vi "Setup - Forrmat Variant Into String.vi"(8 "error in (no error)":errorcluster) -> (0 "error out":errorcluster, 2 "Input String":string, 3 "Refnum":refnum<file>)   [LabVIEW 2009]
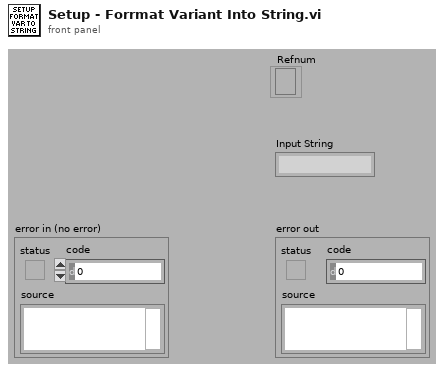
[diagram p1: front panel]
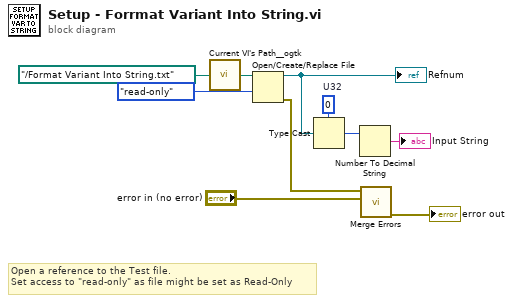
[diagram p0: block diagram]
diagram:
  w7 = u32 0  # U32
  # "Open a reference to the Test file.\nSet access to \"read-only\" as file might be set as Read-Only"
  n1 = call <userlib>:"Current VI's Path__ogtk.vi"("Relative path (.)"=path "../Format Variant Into String.txt" ("file path (use dialog)")) -> ("Current VI's Path (+ Relative)"=w8:path)
  n2 = Open/Create/Replace File(file path (use dialog)=w8, access (0:read/write)=enum16{"read/write", "read-only", "write-only"}."read-only") -> (refnum out=w5:refnum<file>, error out=w2:errorcluster)  [unwired: 4 in, 1 out]
  "Refnum" <- w5
  n3 = Type Cast(type=w7, x=w5) -> (*(type *) &x=w6:u32)
  n4 = Number To Decimal String(number=w6) -> (decimal integer string=→"Input String":string)  [unwired: 1 in]
  n5 = call <vilib>:"Merge Errors.vi"("error in 2 (no error)"="error in (no error)", "error in 1 (no error)"=w2) -> ("error out"=→"error out":errorcluster)  [unwired: 5 in]
